vi "Write.vi"(0 "tdata":bool[](array[boolean]), 1 "tlast":bool, 2 "niInstr AXI4-Stream Writer v1 FPGA in":refnum<class "niInstr AXI4-Stream Writer v1 FPGA.lvclass">, 5 "tstrb":bool[](array[boolean]), 7 "tkeep":bool[](array[boolean]), 9 "input valid":bool, 12 "tuser":bool[](array[boolean])) -> (14 "ready for input":bool)   [LabVIEW 2015, in "niInstr AXI4-Stream Writer v1 FPGA.lvclass"]
doc: "Performs a write operation on the AXI4-Stream Writer.\n\n<B>Input Parameters</B>\n\n<B>tdata</B> is the data to write using the AXI4-Stream Writer.\n\n<B>tlast</B> indicates whether this data is at the boundary of a packet.\n\n<B>niInstr AXI4-Stream Writer v1 FPGA in</B> takes in a reference to the AXI4-Stream Writer from the previous VI.\n\n<B>tstrb</B> is the byte qualifier which indicates whether the content of the associated byte of 'tdata' is a data byte or a position byte.\n\n<B>tkeep</B> is the byte qualifier which indicates whether to process the associated TDATA byte. Bytes associated with a deasserted TKEEP are null bytes and can be removed from the data stream.\n\n<B>input valid</B> indicates whether or not the data on this clock cycle is valid.\n\n<B>tuser</B> is user-defined sideband information that can be transmitted alongside the data stream.\n\n<B>Output Parameters</B>\n\n<B>ready for input</B> indicates whether the bus interface is ready to receive more data."
uses:
  <instrlib>/_niInstr/CLIP Adapters/v1/FPGA/AXI4-Stream/Writer/niInstr AXI4-Stream Writer v1 FPGA.lvclass
  <instrlib>/_niInstr/CLIP Adapters/v1/FPGA/AXI4-Stream/Writer/niInstr AXI4-Stream Writer v1 FPGA.lvclass/niInstr AXI4-Stream Writer v1 FPGA.ctl
  <vilib>/rvi/eio/common/nirviEmuTemplateMethod_errors.vi
  <vilib>/eio/EIONode/EIONode.xnode
  <instrlib>/_niInstr/Basic Elements/v1/FPGA/niInstr Basic Elements v1 FPGA.lvlib
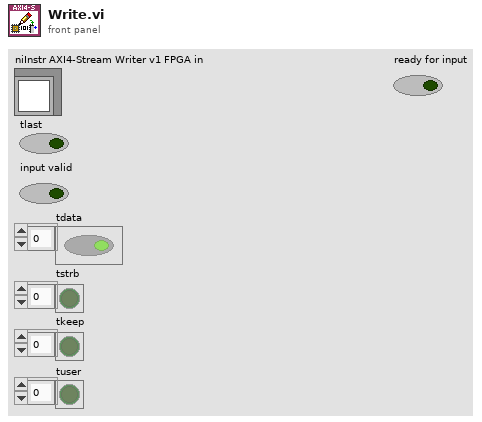
[diagram p1: front panel]
types:
  T1 = cluster{"TDATA Width":i16, "TKEEP Width":i16, "TSTRB Width":i16, "TUSER Width":i16}
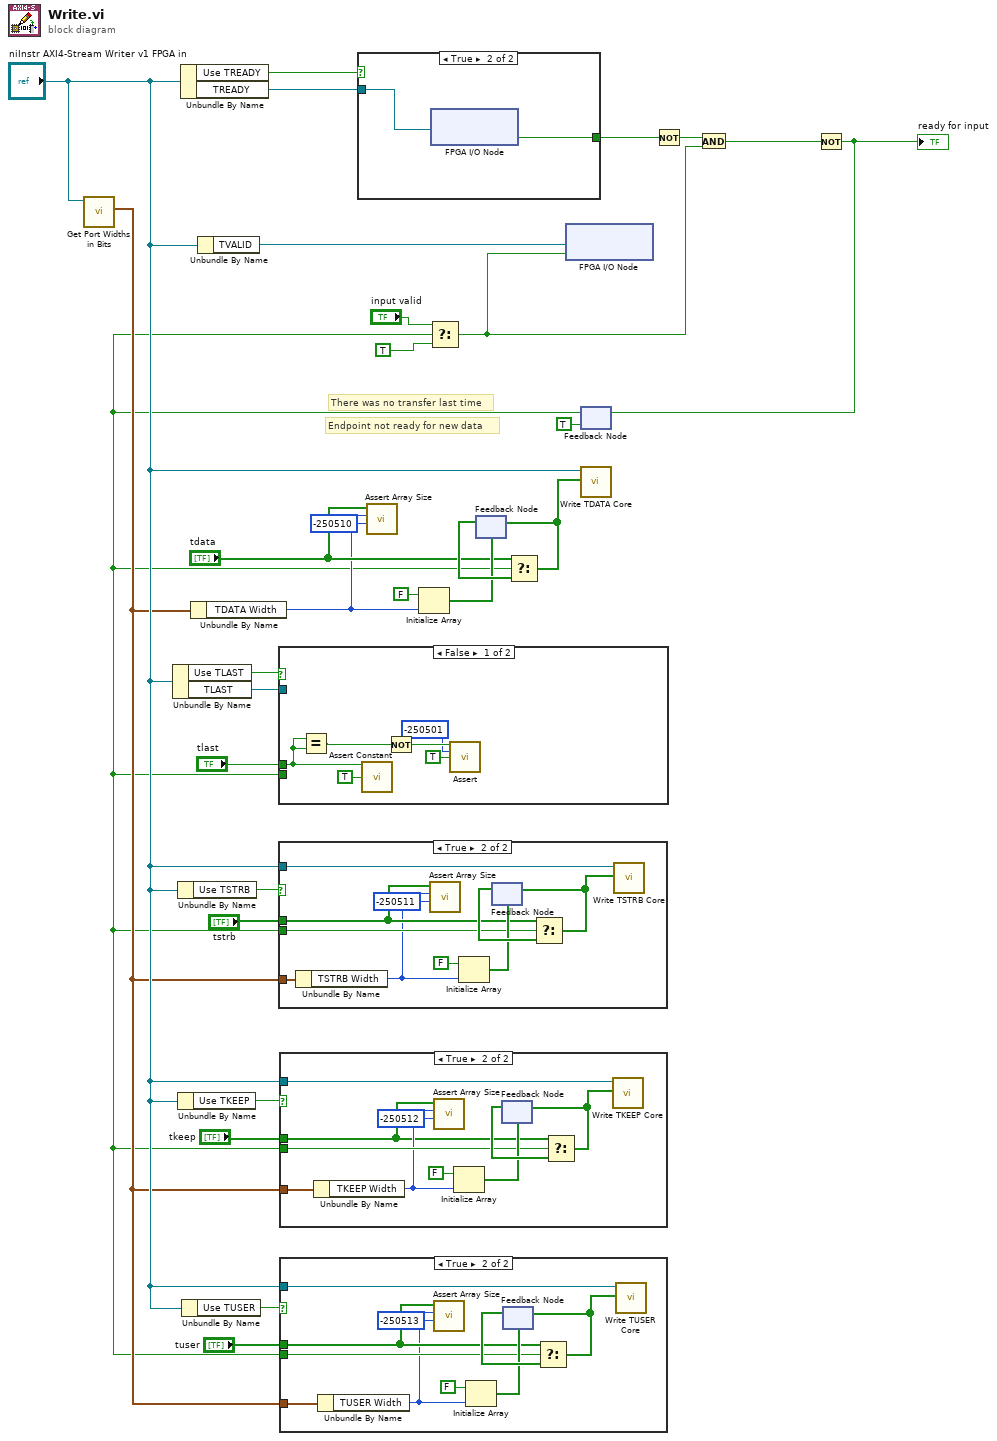
[diagram p0: block diagram]
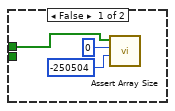
[diagram p2: hidden frame]
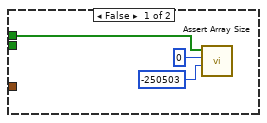
[diagram p3: hidden frame]
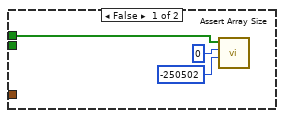
[diagram p4: hidden frame]
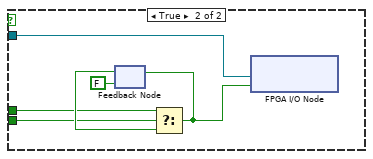
[diagram p5: hidden frame]
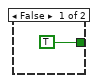
[diagram p6: hidden frame]
diagram:
  # "Endpoint not ready for new data"
  # "There was no transfer last time"
  n1 = call-dynamic "Get Port Widths in Bits.vi"("niInstr AXI4-Stream Writer v1 FPGA in"="niInstr AXI4-Stream Writer v1 FPGA in") -> ("port widths"=w13:T1)  [unwired: 9 in, 1 out]
  n2 = Unbundle By Name("niInstr AXI4-Stream Writer v1 FPGA in") -> ("Use TLAST"=w15:bool, "TLAST"=w27:refnum<k21>)
  n3 = Unbundle By Name("niInstr AXI4-Stream Writer v1 FPGA in") -> ("Use TSTRB"=w14:bool)
  n4 = Unbundle By Name("niInstr AXI4-Stream Writer v1 FPGA in") -> ("Use TKEEP"=w12:bool)
  n5 = Unbundle By Name("niInstr AXI4-Stream Writer v1 FPGA in") -> ("Use TREADY"=w30:bool, "TREADY"=w28:refnum<k21>)
  n6 = Unbundle By Name("niInstr AXI4-Stream Writer v1 FPGA in") -> ("Use TUSER"=w11:bool)
  n7 = Unbundle By Name(w13) -> ("TDATA Width"=w3:i16)
  n8 = Unbundle By Name("niInstr AXI4-Stream Writer v1 FPGA in") -> ("TVALID"=w20:refnum<k21>)
  n9 = case shown="True" w30 {
    tunnel: w28 -> [_ w33]
    tunnel: [TRUE ("I/O Item") w32] -> w24
    frame False {
    }
    frame True {
      n10 = xnode "FPGA I/O Node"("FPGA I/O In"=w33) -> ("I/O Item"=w32:bool)  [unwired: 1 out]
    }
  }
  n11 = call <instrlib>:"Assert Array Size.vi"("error code"=-250510, "size"=w3, "boolean array"="tdata") -> ()  [unwired: 9 in]
  n12 = Initialize Array(FALSE ("TLAST Value"), w3) -> (w16:bool[])
  n13 = feedback #1(w16) -> (w21:bool[])
  n14 = feedback #2(TRUE) -> (w2:bool)
  n15 = case shown="False" w15 {
    tunnel: w27 -> [_ w45]
    tunnel: w2 -> [_ w41]
    tunnel: "tlast" -> [w35 w40]
    frame False {
      n16 = Equal?(x=w35, y=w35) -> (x = y?=w34:bool)
      n17 = call <instrlib>:"Assert Constant.vi"("constant terminal"=w35, "enable show error"=TRUE) -> ()  [unwired: 14 in]
      n18 = Not(x=w34) -> (.not. x?=w38:bool)
      n19 = call <instrlib>:"Assert.vi"("assert"=w38, "error code"=-250501, "enable show error"=TRUE) -> ()  [unwired: 13 in]
    }
    frame True {
      n20 = feedback #3(FALSE ("TLAST Value")) -> (w43:bool)
      n21 = Select(t=w40, s=w41, f=w43) -> (s? t:f=w44:bool)
      n22 = feedback-in #3(w44) -> ()
      n23 = xnode "FPGA I/O Node"("I/O Item"=w44, "FPGA I/O In"=w45) -> ()  [unwired: 1 out]
    }
  }
  n24 = case shown="True" w14 {
    tunnel: "niInstr AXI4-Stream Writer v1 FPGA in" -> [_ w57]
    tunnel: w13 -> [_ w55]
    tunnel: w2 -> [_ w52]
    tunnel: "tstrb" -> [w46 w51]
    frame False {
      n25 = call <instrlib>:"Assert Array Size.vi"("error code"=-250502, "size"=0, "boolean array"=w46) -> ()  [unwired: 9 in]
    }
    frame True {
      n26 = Unbundle By Name(w55) -> ("TSTRB Width"=w50:i16)
      n27 = call <instrlib>:"Assert Array Size.vi"("error code"=-250511, "size"=w50, "boolean array"=w51) -> ()  [unwired: 9 in]
      n28 = Initialize Array(FALSE ("TLAST Value"), w50) -> (w53:bool[])
      n29 = feedback #4(w53) -> (w58:bool[])
      n30 = Select(t=w51, s=w52, f=w58) -> (s? t:f=w54:bool[])
      n31 = feedback-in #4(w54) -> ()
      n32 = call-dynamic "Write TSTRB Core.vi"("value"=w54, "niInstr AXI4-Stream Writer v1 FPGA in"=w57) -> ()  [unwired: 9 in, 1 out]
    }
  }
  n33 = case shown="True" w12 {
    tunnel: "niInstr AXI4-Stream Writer v1 FPGA in" -> [_ w70]
    tunnel: w13 -> [_ w68]
    tunnel: w2 -> [_ w65]
    tunnel: "tkeep" -> [w59 w63]
    frame False {
      n34 = call <instrlib>:"Assert Array Size.vi"("error code"=-250503, "size"=0, "boolean array"=w59) -> ()  [unwired: 9 in]
    }
    frame True {
      n35 = Unbundle By Name(w68) -> ("TKEEP Width"=w64:i16)
      n36 = call <instrlib>:"Assert Array Size.vi"("error code"=-250512, "size"=w64, "boolean array"=w63) -> ()  [unwired: 9 in]
      n37 = Initialize Array(FALSE ("TLAST Value"), w64) -> (w66:bool[])
      n38 = feedback #5(w66) -> (w71:bool[])
      n39 = Select(t=w63, s=w65, f=w71) -> (s? t:f=w67:bool[])
      n40 = feedback-in #5(w67) -> ()
      n41 = call-dynamic "Write TKEEP Core.vi"("value"=w67, "niInstr AXI4-Stream Writer v1 FPGA in"=w70) -> ()  [unwired: 9 in, 1 out]
    }
  }
  n42 = case shown="True" w11 {
    tunnel: "niInstr AXI4-Stream Writer v1 FPGA in" -> [_ w83]
    tunnel: w13 -> [_ w81]
    tunnel: w2 -> [_ w78]
    tunnel: "tuser" -> [w73 w77]
    frame False {
      n43 = call <instrlib>:"Assert Array Size.vi"("error code"=-250504, "size"=0, "boolean array"=w73) -> ()  [unwired: 9 in]
    }
    frame True {
      n44 = Unbundle By Name(w81) -> ("TUSER Width"=w76:i16)
      n45 = call <instrlib>:"Assert Array Size.vi"("error code"=-250513, "size"=w76, "boolean array"=w77) -> ()  [unwired: 9 in]
      n46 = Initialize Array(FALSE ("TLAST Value"), w76) -> (w79:bool[])
      n47 = feedback #6(w79) -> (w84:bool[])
      n48 = Select(t=w77, s=w78, f=w84) -> (s? t:f=w80:bool[])
      n49 = feedback-in #6(w80) -> ()
      n50 = call-dynamic "Write TUSER Core.vi"("value"=w80, "niInstr AXI4-Stream Writer v1 FPGA in"=w83) -> ()  [unwired: 9 in, 1 out]
    }
  }
  n51 = Select(t="input valid", s=w2, f=TRUE) -> (s? t:f=w19:bool)
  n52 = Select(t="tdata", s=w2, f=w21) -> (s? t:f=w5:bool[])
  n53 = feedback-in #1(w5) -> ()
  n54 = xnode "FPGA I/O Node"("I/O Item"=w19, "FPGA I/O In"=w20) -> ()  [unwired: 1 out]
  n55 = call-dynamic "Write TDATA Core.vi"("raw data"=w5, "niInstr AXI4-Stream Writer v1 FPGA in"="niInstr AXI4-Stream Writer v1 FPGA in") -> ()  [unwired: 9 in, 1 out]
  n56 = Not(x=w24) -> (.not. x?=w25:bool)
  n57 = And(x=w25, y=w19) -> (x .and. y?=w26:bool)
  n58 = Not(x=w26) -> (.not. x?=w22:bool)
  "ready for input" <- w22
  n59 = feedback-in #2(w22) -> ()
